vi "短日期时间转长日期格式.vi"(10 "table输入":string(combo), 11 "data":string[][](table)) -> (3 "输出数组":string[][](array[string]))   [LabVIEW 2016, in "数据传输系统.lvlib"]
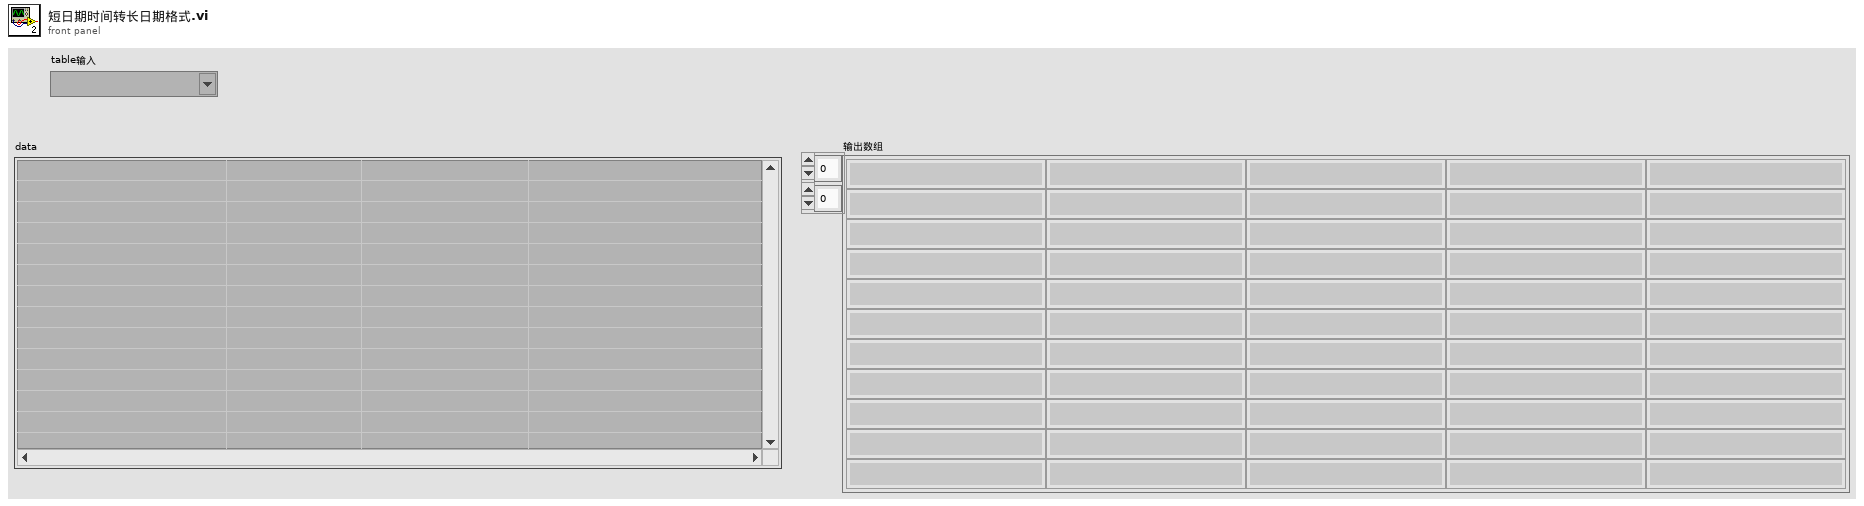
[diagram p1: front panel]
types:
  T1 = typedef "LVDateTimeRec.ctl" = cluster{"秒数的小数部分":dbl, "秒":i32, "分":i32, "时":i32, "日":i32, "月":i32, "年":i32, "天数（周）":i32, "天数（年）":i32, "DST":i32}
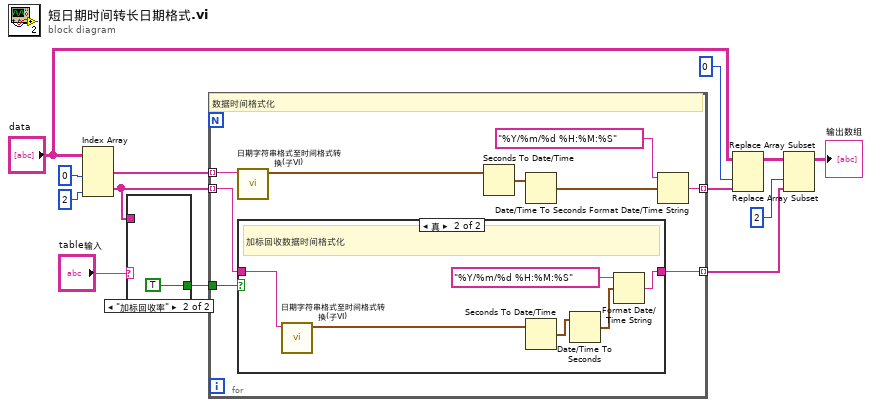
[diagram p0: block diagram]
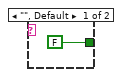
[diagram p3: hidden frame]
diagram:
  n1 = Index Array(array="data", index (col) #1=0 ("禁用的索引 (列)"), index (col) #2=2 ("索引 (列)")) -> (element #1=w2:string[], element #2=w1:string[])  [unwired: 2 in]
  n2 = case shown="\"加标回收率\"" "table输入" {
    tunnel: [FALSE TRUE] -> w3
    tunnel: w1 -> [_ _]
    frame "", Default {
    }
    frame "加标回收率" {
    }
  }
  n3 = for {
    tunnel: [w20] -> w9 mode=indexing
    tunnel: [w19] -> w5 mode=indexing
    tunnel: w3 -> [w18]
    tunnel: w2 -> [w17] mode=indexing
    tunnel: w1 -> [w16] mode=indexing
    # "数据时间格式化"
    n4 = call "日期字符串格式至时间格式转换(子VI).vi"("data[0]"=w17) -> ("time stamp"=w23:timestamp)  [unwired: 10 in]
    n5 = case shown="真" w18 {
      tunnel: [w25 w27] -> w19
      tunnel: w16 -> [w25 w26]
      frame False {
      }
      frame True {
        # "加标回收数据时间格式化"
        n6 = call "日期字符串格式至时间格式转换(子VI).vi"("data[0]"=w26) -> ("time stamp"=w29:timestamp)  [unwired: 10 in]
        n7 = Seconds To Date/Time(time stamp (now)=w29) -> (date time rec=w28:T1)  [unwired: 1 in]
        n8 = Date/Time To Seconds(2:w28) -> (0:w30:timestamp)  [unwired: 1 in]
        n9 = Format Date/Time String(time format string (%c)="%Y/%m/%d %H:%M:%S" ("时间格式字符串(%c)"), seconds (now)=w30) -> (date/time string=w27:string)  [unwired: 1 in]
      }
    }
    n10 = Seconds To Date/Time(time stamp (now)=w23) -> (date time rec=w24:T1)  [unwired: 1 in]
    n11 = Date/Time To Seconds(2:w24) -> (0:w22:timestamp)  [unwired: 1 in]
    n12 = Format Date/Time String(time format string (%c)="%Y/%m/%d %H:%M:%S" ("时间格式字符串(%c)"), seconds (now)=w22) -> (date/time string=w20:string)  [unwired: 1 in]
  }
  n13 = Replace Array Subset(array="data", new element=w9, index (col)=0 ("禁用的索引 (列)")) -> (w6:string[][])  [unwired: 1 in]
  n14 = Replace Array Subset(array=w6, new element=w5, index (col)=2 ("索引 (列)")) -> (→"输出数组":string[][])  [unwired: 1 in]
